vi "Write NumScans.vi"(8 "error in (no error)":errorcluster, 10 "NumScans":i16=-1 caption="Nr Of Scans", 11 "SEDSpectrometer in":refnum<class "FiberSpectrograph.lvclass">) -> (0 "error out":errorcluster, 3 "SEDSpectrometer out":refnum<class "FiberSpectrograph.lvclass">)   [LabVIEW 2016, in "FiberSpectrograph.lvclass"]
uses:
  FiberSpectrograph.lvclass
  FiberSpectrograph.lvclass/FiberSpectrograph.ctl
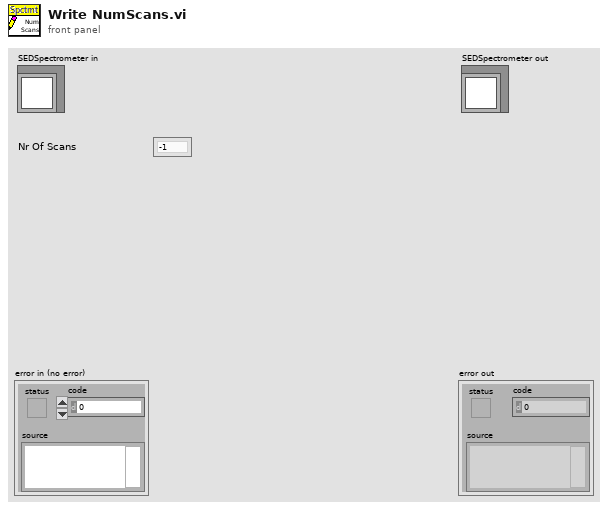
[diagram p1: front panel]
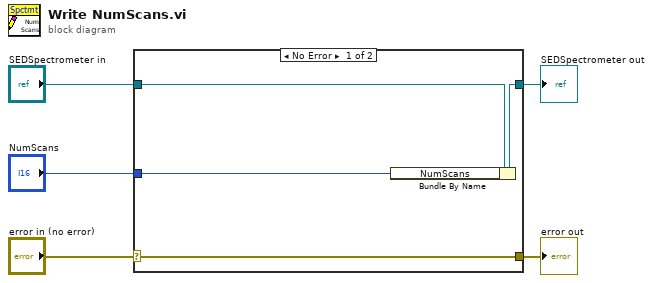
[diagram p0: block diagram]
diagram:
  n1 = case shown="No Error" "error in (no error)" {
    selector: "error in (no error)" -> [w9 w10]
    tunnel: [w9 w10] -> w4
    tunnel: [w7 w11] -> w2
    tunnel: "SEDSpectrometer in" -> [w8 w11]
    tunnel: "NumScans" -> [w6 _]
    frame No Error {
      n2 = Bundle By Name(cluster=w8, "NumScans"=w6) -> (w7:refnum<class "FiberSpectrograph.lvclass">)
    }
    frame Error {
    }
  }
  "error out" <- w4
  "SEDSpectrometer out" <- w2
